vi "R5pHControl.vi"(8 "error constant":errorcluster, 11 "LabVIEW Web Service":refnum<class "Web Service.lvclass">) -> ()   [LabVIEW 2016]
uses:
  <vilib>/wsapi/Web Service.lvclass
  Controls/pH_SetParams Standard.ctl
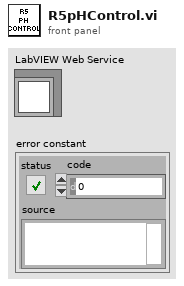
[diagram p1: front panel]
types:
  T1 = typedef "pH_SetParams Standard.ctl" = cluster{"Set Point":dbl, "Tolerance":dbl, "Pump Time On, secs":dbl}
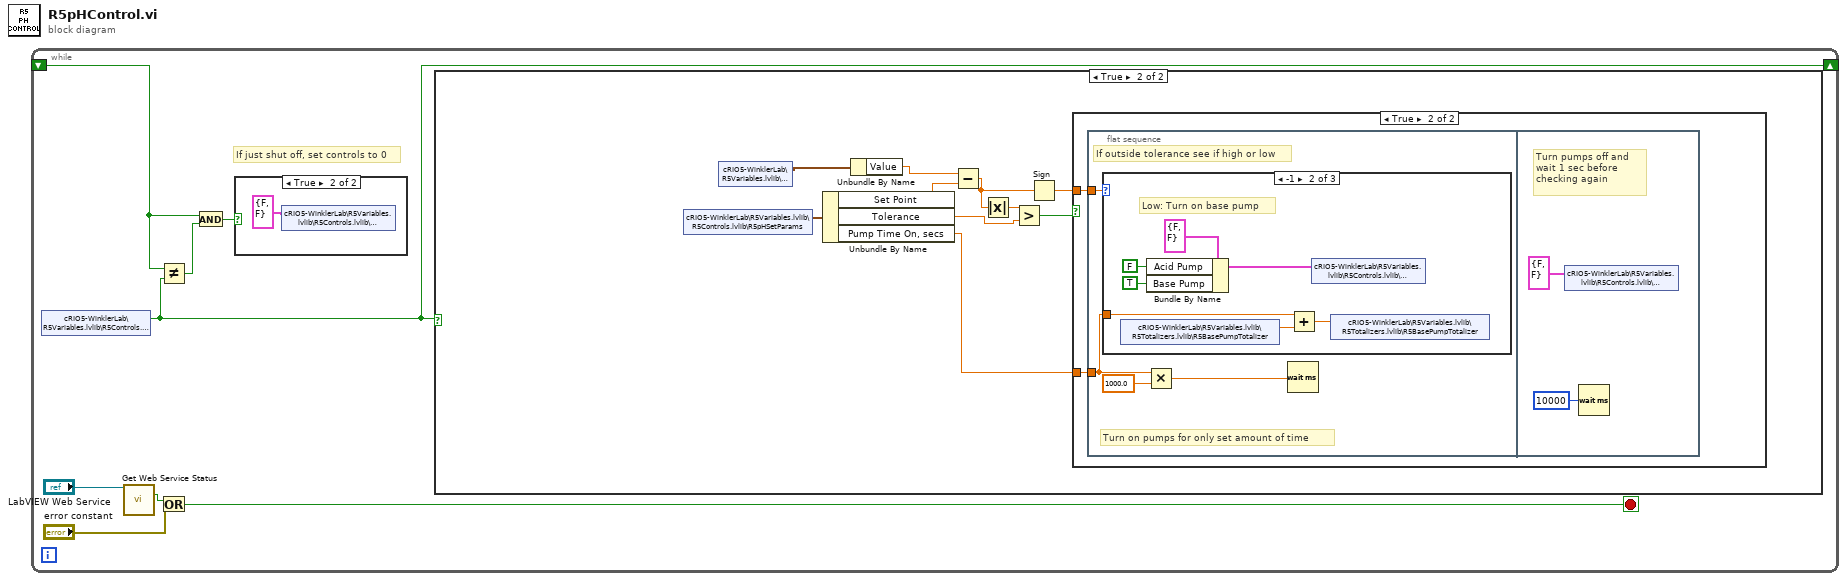
[diagram p0: block diagram]
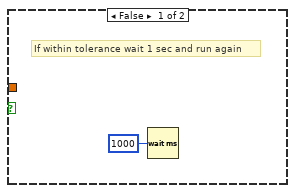
[diagram p4: hidden frame]
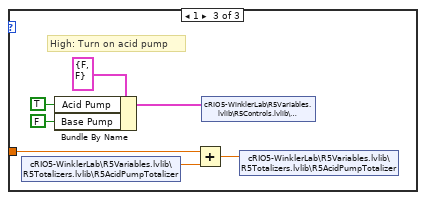
[diagram p6: hidden frame]
diagram:
  n1 = while {
    shift-right: [w1] -> _
    shift-left: _ -> [w3]
    stop <- w5 stop-if-true
    # "If just shut off, set controls to 0"
    n2 = shared-variable "cRIO5-WinklerLab\\R5Variables.lvlib\\R5Controls.lvlib\\R5pHSwitch"() -> (w1:bool)  [unwired: 1 in, 1 out]
    n3 = call <vilib>:"Get Web Service Status.vi"("LabVIEW Web Service"="LabVIEW Web Service") -> ("service stopping?"=w8:bool)  [unwired: 12 in, 2 out]
    n4 = Not Equal?(x=w3, y=w1) -> (x != y?=w4:bool)
    n5 = Or(x=w8, y="error constant") -> (x .or. y?=w5:bool)
    n6 = And(x=w3, y=w4) -> (x .and. y?=w2:bool)
    n7 = case shown="True" w2 {
      frame False {
      }
      frame True {
        n8 = shared-variable "cRIO5-WinklerLab\\R5Variables.lvlib\\R5Controls.lvlib\\R5pHManual"(cluster{"Acid Pump":bool, "Base Pump":bool} {"Acid Pump"=FALSE, "Base Pump"=FALSE} ("R1pHManual")) -> ()  [unwired: 1 in, 1 out]
      }
    }
    n9 = case shown="True" w1 {
      frame False {
        # "Don't do anything if control is off"
      }
      frame True {
        n10 = shared-variable "cRIO5-WinklerLab\\R5Variables.lvlib\\R5Controls.lvlib\\R5pHSetParams"() -> (w10:T1)  [unwired: 1 in, 1 out]
        n11 = shared-variable "cRIO5-WinklerLab\\R5Variables.lvlib\\R5Signals.lvlib\\R5pH"() -> (w11:cluster{"Signal":dbl, "Value":dbl})  [unwired: 1 in, 1 out]
        n12 = Unbundle By Name(w10) -> ("Set Point"=w18:dbl, "Tolerance"=w16:dbl, "Pump Time On, secs"=w12:dbl)
        n13 = Unbundle By Name(w11) -> ("Value"=w19:dbl)
        n14 = Subtract(x=w19, y=w18) -> (x-y=w14:dbl)
        n15 = Absolute Value(x=w14) -> (abs(x)=w17:dbl)
        n16 = Greater?(x=w17, y=w16) -> (0:w15:bool)
        n17 = Sign(1:w14) -> (0:w13:dbl)
        n18 = case shown="True" w15 {
          tunnel: w13 -> [_ w22]
          tunnel: w12 -> [_ w21]
          frame False {
            # "If within tolerance wait 1 sec and run again"
            n19 = Wait (ms)(milliseconds to wait=u32 1000) -> ()  [unwired: 1 out]
          }
          frame True {
            n20 = flat-sequence {
              tunnel: w22 -> [w26]
              tunnel: w21 -> [w23]
              frame #0 {
                # "Turn on pumps for only set amount of time"
                # "If outside tolerance see if high or low"
                n21 = case shown="-1" w26 {
                  tunnel: w23 -> [_ w30 w37]
                  frame 0, Default {
                    # "Unless tolerance is 0 this code\nshouldn't be accesible"
                  }
                  frame -1 {
                    # "Low: Turn on base pump"
                    n22 = shared-variable "cRIO5-WinklerLab\\R5Variables.lvlib\\R5Totalizers.lvlib\\R5BasePumpTotalizer"() -> (w28:dbl)  [unwired: 1 in, 1 out]
                    n23 = Bundle By Name(cluster=cluster{"Acid Pump":bool, "Base Pump":bool} {"Acid Pump"=FALSE, "Base Pump"=FALSE} ("R1pHManual"), "Acid Pump"=FALSE, "Base Pump"=TRUE) -> (w27:cluster{"Acid Pump":bool, "Base Pump":bool})
                    n24 = Add(x=w30, y=w28) -> (x+y=w29:dbl)
                    n25 = shared-variable "cRIO5-WinklerLab\\R5Variables.lvlib\\R5Controls.lvlib\\R5pHManual"(w27) -> ()  [unwired: 1 in, 1 out]
                    n26 = shared-variable "cRIO5-WinklerLab\\R5Variables.lvlib\\R5Totalizers.lvlib\\R5BasePumpTotalizer"(w29) -> ()  [unwired: 1 in, 1 out]
                  }
                  frame 1 {
                    # "High: Turn on acid pump"
                    n27 = shared-variable "cRIO5-WinklerLab\\R5Variables.lvlib\\R5Totalizers.lvlib\\R5AcidPumpTotalizer"() -> (w34:dbl)  [unwired: 1 in, 1 out]
                    n28 = Bundle By Name(cluster=cluster{"Acid Pump":bool, "Base Pump":bool} {"Acid Pump"=FALSE, "Base Pump"=FALSE} ("R1pHManual"), "Acid Pump"=TRUE, "Base Pump"=FALSE) -> (w36:cluster{"Acid Pump":bool, "Base Pump":bool})
                    n29 = Add(x=w37, y=w34) -> (x+y=w35:dbl)
                    n30 = shared-variable "cRIO5-WinklerLab\\R5Variables.lvlib\\R5Controls.lvlib\\R5pHManual"(w36) -> ()  [unwired: 1 in, 1 out]
                    n31 = shared-variable "cRIO5-WinklerLab\\R5Variables.lvlib\\R5Totalizers.lvlib\\R5AcidPumpTotalizer"(w35) -> ()  [unwired: 1 in, 1 out]
                  }
                }
                n32 = Multiply(x=w23, y=1000.0) -> (x*y=w24:dbl)
                n33 = Wait (ms)(milliseconds to wait=w24) -> ()  [unwired: 1 out]
              }
              frame #1 {
                # "Turn pumps off and \nwait 1 sec before\nchecking again"
                n34 = shared-variable "cRIO5-WinklerLab\\R5Variables.lvlib\\R5Controls.lvlib\\R5pHManual"(cluster{"Acid Pump":bool, "Base Pump":bool} {"Acid Pump"=FALSE, "Base Pump"=FALSE} ("R1pHManual")) -> ()  [unwired: 1 in, 1 out]
                n35 = Wait (ms)(milliseconds to wait=u32 10000) -> ()  [unwired: 1 out]
              }
            }
          }
        }
      }
    }
  }
